vi "Create Startup CDF (Components).vi"(3 "Application Path":path, 5 "Device Class":string, 6 "Dependencies":T1[](array[typedef]) {"component type" items=["standard", "hidden", "system", "unknown", "startup", "image"]}, 7 "Operating System":string, 8 "error in (no error)":errorcluster, 9 "Files":path[](array[path]), 10 "Application Info":T1={"title"="", "description"="", "ID"="", "version"="", "component type"=4} {"component type" items=["standard", "hidden", "system", "unknown", "startup", "image"]}, 11 "CDF Location":path) -> (0 "error out":errorcluster)   [LabVIEW 2014, in "nisyscfg.lvlib"]
uses:
  nisyscfg.lvlib
  Software 1.2.ctl
  Component Type.ctl
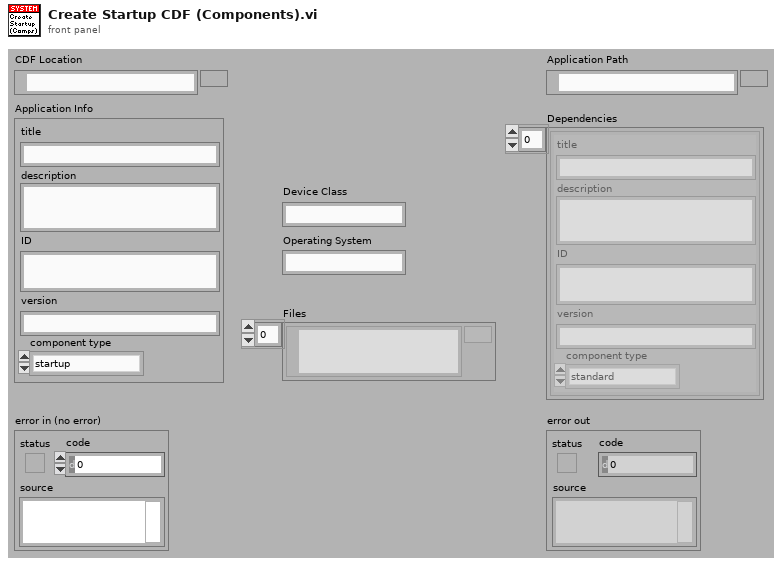
[diagram p1: front panel]
types:
  T1 = typedef "nisyscfg.lvlib/Software 1.2.ctl" = cluster{"title":string, "description":string, "ID":string, "version":string, "component type":T2}
  T2 = typedef "nisyscfg.lvlib/Component Type.ctl" = u32
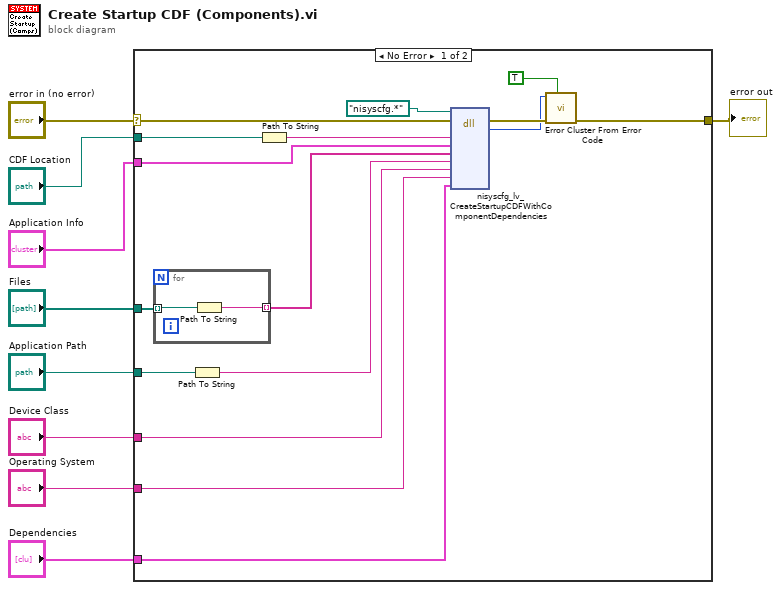
[diagram p0: block diagram]
diagram:
  n1 = case shown="No Error" "error in (no error)" {
    selector: "error in (no error)" -> [w21 w28]
    tunnel: [w20 w28] -> w8
    tunnel: "CDF Location" -> [w19 _]
    tunnel: "Application Info" -> [w14 _]
    tunnel: "Files" -> [w13 _]
    tunnel: "Device Class" -> [w17 _]
    tunnel: "Operating System" -> [w16 _]
    tunnel: "Dependencies" -> [w15 _]
    tunnel: "Application Path" -> [w11 _]
    frame No Error {
      n2 = for {
        tunnel: w13 -> [w27] mode=indexing
        tunnel: [w26] -> w12 mode=indexing
        n3 = Path To String(path=w27) -> (string=w26:string)
      }
      n4 = Path To String(path=w11) -> (string=w10:string)
      n5 = Path To String(path=w19) -> (string=w18:string)
      n6 = dll-call lib="C:/projects/MAX/components/apis/trunk/5.0/objects/scs_nisyscfg_library_dynamic/win32U/i386/msvc90/debug/nisyscfg.dll" fn="nisyscfg_lv_CreateStartupCDFWithComponentDependencies" label="CreateStartupCDFWithComponentDependencies"(path in=path "nisyscfg.*", error in=w21, "cdfLocation"=w18, "applicationInfo"=w14, "files"=w12, "applicationPath"=w10, "deviceClass"=w17, "operatingSystem"=w16, "dependencies"=w15) -> (error out=w25:errorcluster, "result"=w24:i32)  [unwired: 8 in, 1 out]
      n7 = call "Error Cluster From Error Code.vi"("show call chain? (False)"=TRUE, "error in (no error)"=w25, "error code (0)"=w24) -> ("error out"=w20:errorcluster)  [unwired: 6 in]
    }
    frame Error {
    }
  }
  "error out" <- w8
